vi "Test Assert Properties.vi"(8 "error in (no error)":errorcluster) -> (0 "error out":errorcluster)   [LabVIEW 2013]
doc: "This example demonstrates how to create a test suite with multiple inner test cases."
uses:
  classes/Test/Test.lvclass
  classes/Assert/Assert.lvclass
  classes/Properties/Properties.lvclass
panel:
  # "See block diagram"
  # "This Test intentionally fails"
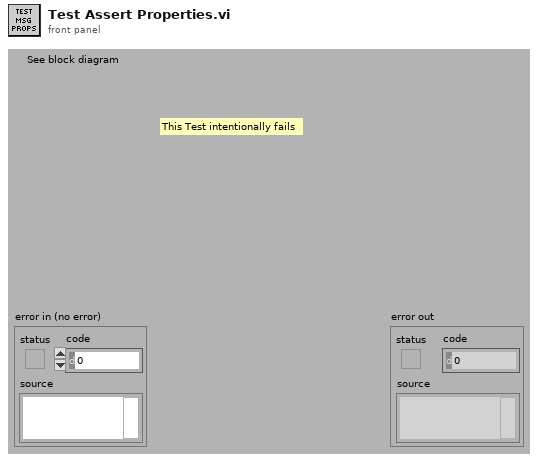
[diagram p1: front panel]
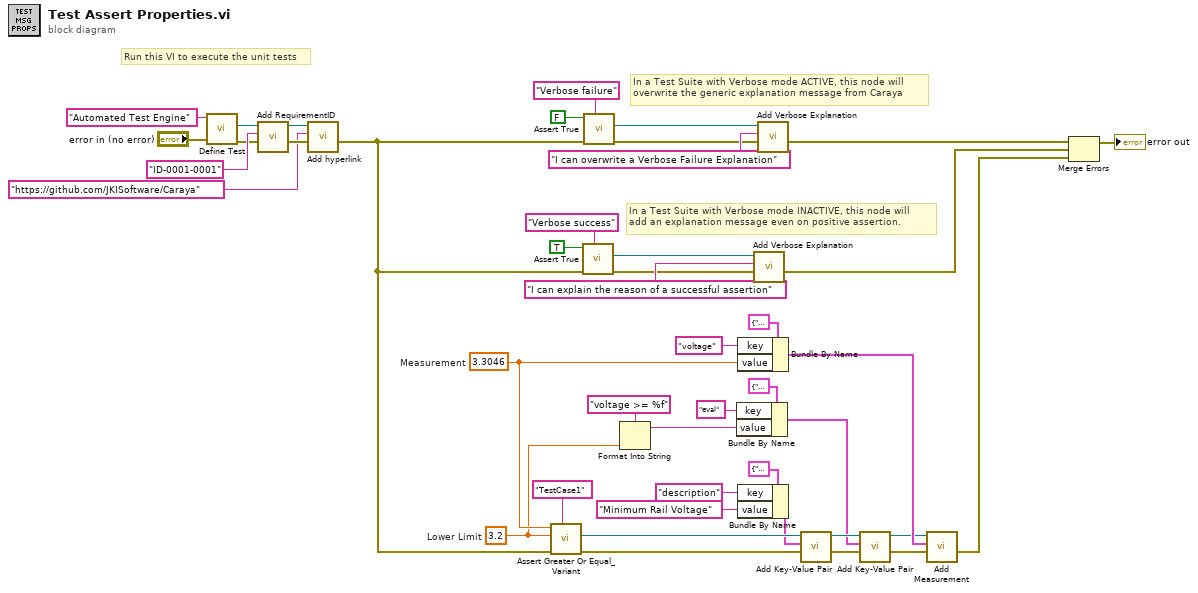
[diagram p0: block diagram]
diagram:
  w24 = 3.3046  # Measurement
  w10 = 3.2  # Lower Limit
  # "In a Test Suite with Verbose mode INACTIVE, this node will\nadd an explanation message even on positive assertion."
  # "In a Test Suite with Verbose mode ACTIVE, this node will\noverwrite the generic explanation message from Caraya"
  # "Run this VI to execute the unit tests"
  n1 = call "Define Test.vi"("error in (no error)"="error in (no error)", "Label (VI Title)"="Automated Test Engine") -> ("error out"=w19:errorcluster, "Properties.Test"=w20:refnum<class "Properties.Test.lvclass">)  [unwired: 8 in]
  n2 = call "Add RequirementID.vi"("error in (no error)"=w19, "Requirement ID"="ID-0001-0001" ("Label"), "Properties"=w20) -> ("error out"=w13:errorcluster, "Properties"=w14:refnum<class "Properties.Test.lvclass">)  [unwired: 7 in]
  n3 = call "Add hyperlink.vi"("error in (no error)"=w13, "URL"="https://github.com/JKISoftware/Caraya" ("Label"), "Properties"=w14) -> ("error out"=w12:errorcluster)  [unwired: 7 in, 1 out]
  n4 = call "Assert Greater Or Equal_Variant.vi"("Label"="TestCase1", "error in (no error)"=w12, "Y"=w10, "X"=w24) -> ("error out"=w30:errorcluster, "Properties.Assert"=w32:refnum<class "Properties.Assert.lvclass">)  [unwired: 6 in]
  n5 = call "Assert True.vi"("Label"="Verbose success", "error in (no error)"=w12, "True?"=TRUE) -> ("error out"=w18:errorcluster, "Properties"=w39:refnum<class "Properties.Assert.lvclass">)  [unwired: 7 in]
  n6 = call "Assert True.vi"("Label"="Verbose failure", "error in (no error)"=w12, "True?"=FALSE) -> ("error out"=w16:errorcluster, "Properties"=w35:refnum<class "Properties.Assert.lvclass">)  [unwired: 7 in]
  n7 = Format Into String(format string="voltage >= %f", w10) -> (resulting string=w4:string)  [unwired: 2 in, 1 out]
  n8 = Bundle By Name(cluster=cluster{"key":string, "value":variant} {"key"="", "value"=variant} ("entry"), "key"="eval", "value"=w4) -> (w2:cluster{"key":string, "value":variant})
  n9 = Bundle By Name(cluster=cluster{"key":string, "value":variant} {"key"="", "value"=variant} ("entry"), "key"="voltage", "value"=w24) -> (w23:cluster{"key":string, "value":variant})
  n10 = Bundle By Name(cluster=cluster{"key":string, "value":variant} {"key"="", "value"=variant} ("entry"), "key"="description", "value"="Minimum Rail Voltage" ("Label")) -> (w28:cluster{"key":string, "value":variant})
  n11 = call "Add Verbose Explanation.vi"("error in (no error)"=w18, "Verbose Explanation"="I can explain the reason of a successful assertion" ("Label"), "Properties"=w39) -> ("error out"=w17:errorcluster)  [unwired: 7 in, 1 out]
  n12 = call "Add Verbose Explanation.vi"("error in (no error)"=w16, "Verbose Explanation"="I can overwrite a Verbose Failure Explanation" ("Label"), "Properties"=w35) -> ("error out"=w15:errorcluster)  [unwired: 7 in, 1 out]
  n13 = call "Add Key-Value Pair.vi"("error in (no error)"=w30, "entry"=w28, "Properties in"=w32) -> ("error out"=w8:errorcluster, "Properties out"=w6:refnum<class "Properties.Assert.lvclass">)  [unwired: 7 in]
  n14 = call "Add Key-Value Pair.vi"("error in (no error)"=w8, "entry"=w2, "Properties in"=w6) -> ("error out"=w7:errorcluster, "Properties out"=w5:refnum<class "Properties.Assert.lvclass">)  [unwired: 7 in]
  n15 = call "Add Measurement.vi"("error in (no error)"=w7, "entry"=w23, "Properties"=w5) -> ("error out"=w22:errorcluster)  [unwired: 7 in, 1 out]
  n16 = Merge Errors(w15, w17, w22) -> (→"error out":errorcluster)
